vi "Gulton_check_reply.vi"(3 "Port Name":string, 4 "Channel Name":string, 5 "Write String":string="L1M?*") -> (0 "Comment out":string, 2 "Read":string)   [LabVIEW 2010]
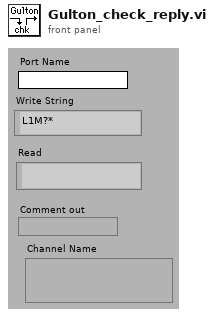
[diagram p1: front panel]
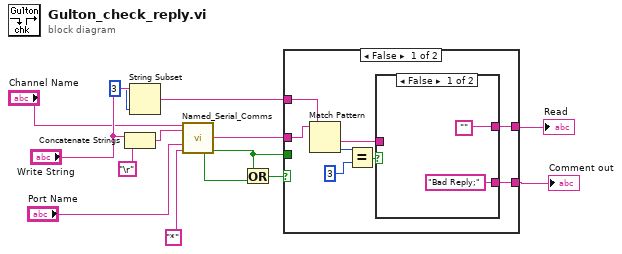
[diagram p0: block diagram]
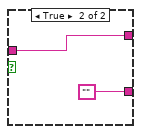
[diagram p2: hidden frame]
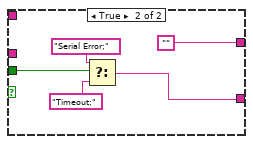
[diagram p3: hidden frame]
diagram:
  n1 = Concatenate Strings("Write String", "\r") -> (w14:string)
  n2 = String Subset(string="Write String", length (rest)=3 ("length")) -> (substring=w4:string)  [unwired: 1 in]
  n3 = call "Named_Serial_Comms.vi"("Channel Name"="Channel Name", "Write String"=w14, "Port Name"="Port Name", "Term Grep"="*" ("Reply Terminator")) -> ("Read"=w13:string, "Timed out"=w10:bool, "Serial Error"=w8:bool)  [unwired: 8 in, 1 out]
  n4 = Or(x=w8, y=w10) -> (x .or. y?=w9:bool)
  n5 = case shown="False" w9 {
    tunnel: w13 -> [w22 _]
    tunnel: [w15 w30] -> w12
    tunnel: [w17 ""] -> w11
    tunnel: w8 -> [_ w31]
    tunnel: w4 -> [w21 _]
    frame False {
      n6 = Match Pattern(string=w22, regular expression=w21) -> (after substring=w16:string, offset past match=w20:i32)  [unwired: 1 in, 2 out]
      n7 = Equal?(x=w20, y=3) -> (x = y?=w18:bool)
      n8 = case shown="False" w18 {
        tunnel: ["" w26] -> w17
        tunnel: w16 -> [_ w26]
        tunnel: ["Bad Reply;" ""] -> w15
        frame False {
        }
        frame True {
        }
      }
    }
    frame True {
      n9 = Select(t="Serial Error;", s=w31, f="Timeout;") -> (s? t:f=w30:string)
    }
  }
  "Read" <- w11
  "Comment out" <- w12
